vi "Find Tests.vi"(8 "error in (no error)":errorcluster, 10 "Project or Class Path":path, 11 "Execution UI In":refnum<class "Execution UI.lvclass">) -> (0 "error out":errorcluster, 3 "Execution UI Out":refnum<class "Execution UI.lvclass">)   [LabVIEW 2020, in "Execution UI.lvclass"]
uses:
  Execution UI.lvclass
  Execution UI.lvclass/Execution UI.ctl
  API/LUnit Test Suite/LUnit Test Suite.lvclass
  Framework/Test Finder/Test Finder.lvclass
  Result Model/Result Model.lvclass
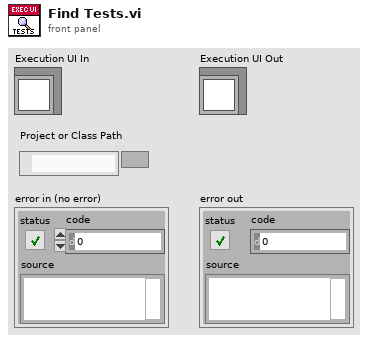
[diagram p1: front panel]
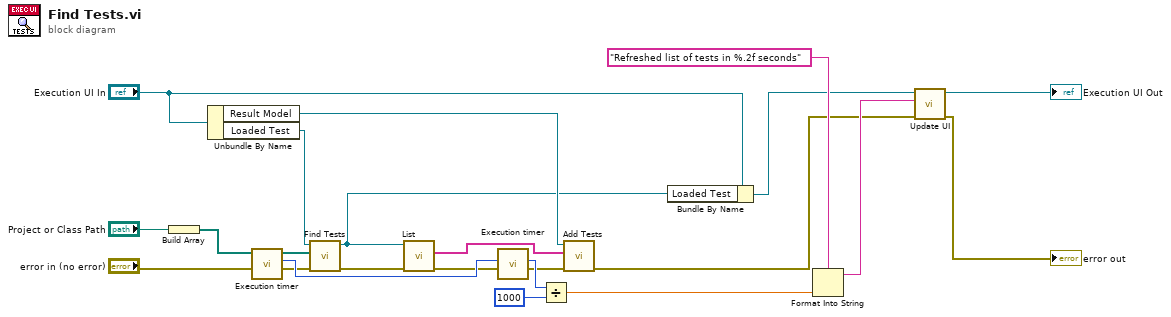
[diagram p0: block diagram]
diagram:
  n1 = Build Array("Project or Class Path") -> (w12:path[])
  n2 = Unbundle By Name("Execution UI In") -> ("Result Model"=w5:refnum<class "Result Model.lvclass">, "Loaded Test"=w1:refnum<class "LUnit Test Suite.lvclass">)
  n3 = call "Execution timer.vi"("error in (no error)"="error in (no error)") -> ("error out"=w15:errorcluster, "Current or Duration [ms]"=w22:u32)  [unwired: 9 in]
  n4 = call "Find Tests.vi"("error in (no error)"=w15, "File Paths"=w12, "LUnit Test Suite"=w1) -> ("error out"=w14:errorcluster, "LUnit Test Suite"=w2:refnum<class "LUnit Test Suite.lvclass">)  [unwired: 7 in]
  n5 = call-dynamic "List.vi"("error in (no error)"=w14, "LUnit Test Suite In"=w2) -> ("error out"=w10:errorcluster, "List of Runnables"=w7:string[])  [unwired: 8 in]
  n6 = call "Execution timer.vi"("error in (no error)"=w10, "millisecond timer value"=w22) -> ("error out"=w4:errorcluster, "Current or Duration [ms]"=w20:u32)  [unwired: 8 in]
  n7 = Divide(x=w20, y=u32 1000) -> (x/y=w21:dbl)
  n8 = call "Add Tests.vi"("error in (no error)"=w4, "Tests"=w7, "Result Model In"=w5) -> ("error out"=w3:errorcluster)  [unwired: 8 in]
  n9 = Bundle By Name(cluster="Execution UI In", "Loaded Test"=w2) -> (w11:refnum<class "Execution UI.lvclass">)
  n10 = Format Into String(format string="Refreshed list of tests in %.2f seconds" ("Status"), w21) -> (resulting string=w17:string)  [unwired: 2 in, 1 out]
  n11 = call "Update UI.vi"("error in (no error)"=w3, "Status"=w17, "Execution UI In"=w11) -> ("error out"=→"error out":errorcluster, "Execution UI Out"=→"Execution UI Out":refnum<class "Execution UI.lvclass">)  [unwired: 7 in]
